vi "Log_WriteLog.vi"(4 "Additional text":string, 6 "All read":string, 8 "error in (no error)":errorcluster, 9 "Response":string, 10 "Command":string, 11 "Log in":refnum<class "Log.lvclass">) -> (0 "error out":errorcluster, 3 "Log out":refnum<class "Log.lvclass">)   [LabVIEW 2024, in "Log.lvclass"]
uses:
  Log.lvclass
  Log.lvclass/Log.ctl
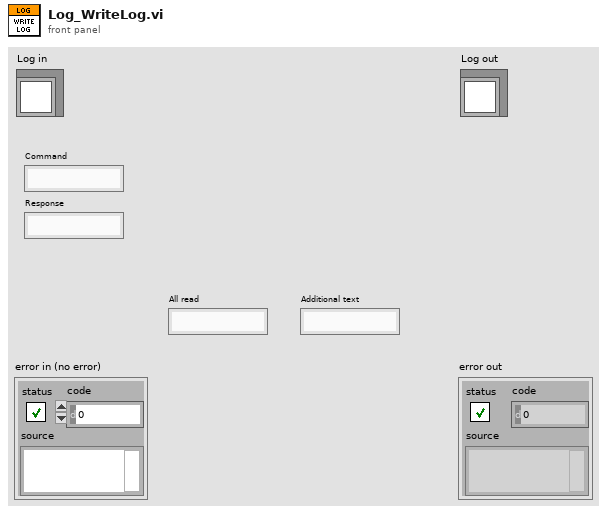
[diagram p1: front panel]
types:
  T1 = enum16{"open", "replace", "create", "open or create", "replace or create", "replace or create with confirmation"}
  T2 = typedef "LVDateTimeRec.ctl" = cluster{"fractional second":dbl, "second":i32, "minute":i32, "hour":i32, "day of month":i32, "month":i32, "year":i32, "day of week":i32, "day of year":i32, "DST":i32}
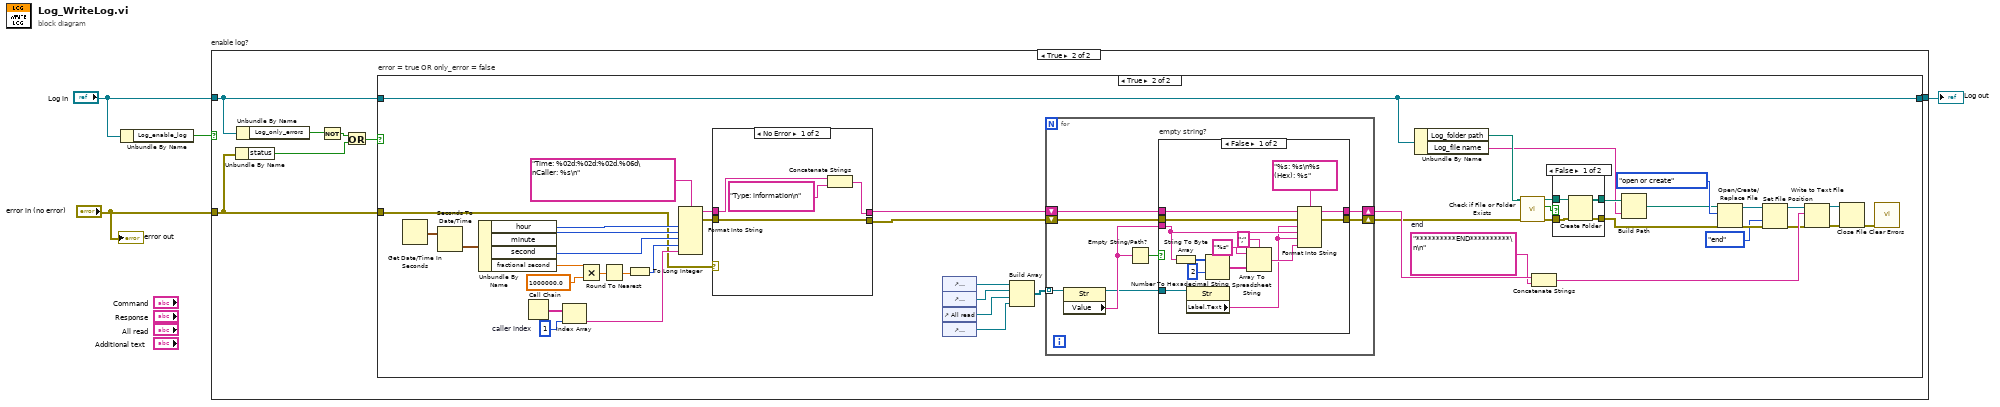
[diagram p0: block diagram]
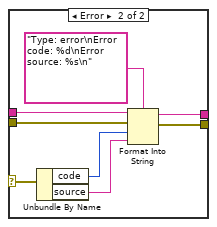
[diagram p6: hidden frame]
diagram:
  n1 = Unbundle By Name("Log in") -> ("Log_enable_log"=w2:bool)
  n2 = case "enable log?" shown="True" w2 {
    tunnel: [w5 w12] -> w4
    tunnel: "Log in" -> [w5 w11]
    tunnel: "error in (no error)" -> [_ w6]
    frame False {
    }
    frame True {
      n3 = Unbundle By Name(w6) -> ("status"=w8:bool)
      n4 = Unbundle By Name(w11) -> ("Log_only_errors"=w10:bool)
      n5 = Not(x=w10) -> (.not. x?=w9:bool)
      n6 = Or(x=w9, y=w8) -> (x .or. y?=w7:bool)
      n7 = case "error = true OR only_error = false" shown="True" w7 {
        tunnel: [w13 w31] -> w12
        tunnel: w11 -> [w13 w31]
        tunnel: w6 -> [_ w41]
        frame False {
        }
        frame True {
          w44 = "**********END**********\n\n"  # end
          w59 = 1  # caller index
          n8 = Get Date/Time In Seconds() -> (seconds since 1Jan1904=w55:timestamp)
          n9 = Seconds To Date/Time(time stamp (now)=w55) -> (date time rec=w47:T2)  [unwired: 1 in]
          n10 = Unbundle By Name(w47) -> ("hour"=w48:i32, "minute"=w49:i32, "second"=w50:i32, "fractional second"=w51:dbl)
          n11 = Call Chain() -> (call chain=w56:string[])
          n12 = Index Array(array=w56, index=w59) -> (element=w46:string)
          n13 = Multiply(x=w51, y=1000000.0) -> (x*y=w52:dbl)
          n14 = Round To Nearest(number=w52) -> (nearest integer value=w53:dbl)
          n15 = To Long Integer(number=w53) -> (32bit integer=w54:i32)
          n16 = Format Into String(format string="Time: %02d:%02d:%02d.%06d\nCaller: %s\n", w48, w49, w50, w54, w46) -> (resulting string=w43:string, error out=w42:errorcluster)  [unwired: 2 in]
          n17 = case shown="No Error" w41 {
            selector: w41 -> [_ w98]
            tunnel: w43 -> [w92 w101]
            tunnel: w42 -> [w93 w100]
            tunnel: [w90 w95] -> w39
            tunnel: [w93 w94] -> w40
            frame No Error {
              n18 = Concatenate Strings(w92, "Type: information\n") -> (w90:string)
            }
            frame Error {
              n19 = Unbundle By Name(w98) -> ("code"=w97:i32, "source"=w96:string)
              n20 = Format Into String(format string="Type: error\nError code: %d\nError source: %s\n", initial string=w101, error in=w100, w97, w96) -> (resulting string=w95:string, error out=w94:errorcluster)
            }
          }
          n21 = control-ref of="Command"() -> (w29:refnum<vi>)
          n22 = control-ref of="Response"() -> (w28:refnum<vi>)
          n23 = control-ref of="All read"() -> (w27:refnum<vi>)
          n24 = control-ref of="Additional text"() -> (w26:refnum<vi>)
          n25 = Build Array(w29, w28, w27, w26) -> (w30:refnum<vi>[])
          n26 = for {
            shift-right: [w63] -> w32
            shift-left: w40 -> [w65]
            shift-right: [w67] -> w45
            shift-left: w39 -> [w64]
            tunnel: w30 -> [w62] mode=indexing
            n27 = property class="Str"(reference=w62) -> (reference out=w60:refnum<vi>, "Value"=w61:string)  [unwired: 1 in, 1 out]
            n28 = Empty String/Path?(string/path=w61) -> (empty?=w66:bool)
            n29 = case "empty string?" shown="False" w66 {
              tunnel: w65 -> [w81 w82]
              tunnel: w64 -> [w80 w83]
              tunnel: [w78 w82] -> w63
              tunnel: [w77 w83] -> w67
              tunnel: w61 -> [w76 _]
              tunnel: w60 -> [w69 _]
              frame False {
                n30 = String To Byte Array(string=w76) -> (unsigned byte array=w75:u8[])
                n31 = property class="Str"(reference=w69) -> ("Label.Text"=w68:string)  [unwired: 1 in, 2 out]
                n32 = Number To Hexadecimal String(1:i16 2 ("width (-)"), 2:w75) -> (0:w73:string[])
                n33 = Array To Spreadsheet String(delimiter (Tab)=";", array=w73, 3:"%s" ("format string")) -> (spreadsheet string=w70:string)
                n34 = Format Into String(format string="%s: %s\n%s (Hex): %s", initial string=w80, error in=w81, w68, w76, w68, w70) -> (resulting string=w77:string, error out=w78:errorcluster)
              }
              frame True {
              }
            }
          }
          n35 = Unbundle By Name(w31) -> ("Log_folder path"=w34:path, "Log_file name"=w33:string)
          n36 = call <vilib>:"Check if File or Folder Exists.vi"("error in (no error)"=w32, "path"=w34) -> ("error out"=w38:errorcluster, "file or folder exists?"=w36:bool, "dup path"=w37:path)  [unwired: 7 in]
          n37 = Concatenate Strings(w45, w44) -> (w25:string)
          n38 = case shown="False" w36 {
            tunnel: w37 -> [w87 w89]
            tunnel: w38 -> [w86 w88]
            tunnel: [w85 w88] -> w22
            tunnel: [w84 w89] -> w35
            frame False {
              n39 = Create Folder(path (use dialog)=w87, error in=w86) -> (created path=w84:path, error out=w85:errorcluster)  [unwired: 1 in, 1 out]
            }
            frame True {
            }
          }
          n40 = Build Path(base path=w35, name or relative path=w33) -> (appended path=w23:path)
          n41 = Open/Create/Replace File(file path (use dialog)=w23, error in=w22, operation (0:open)=T1."open or create") -> (refnum out=w17:refnum<file>, error out=w18:errorcluster)  [unwired: 3 in, 1 out]
          n42 = Set File Position(refnum=w17, from (0:start)=enum16{"start", "end", "current"}."end", error in=w18) -> (refnum out=w15:refnum<file>, error out=w14:errorcluster)  [unwired: 1 in]
          n43 = Write to Text File(file (use dialog)=w15, text=w25, error in=w14) -> (refnum out=w19:refnum<file>, error out=w20:errorcluster)  [unwired: 1 in, 1 out]
          n44 = Close File(refnum=w19, error in=w20) -> (error out=w21:errorcluster)  [unwired: 1 out]
          n45 = call <vilib>:"Clear Errors.vi"("error in (no error)"=w21) -> ()  [unwired: 5 in, 2 out]
        }
      }
    }
  }
  "Log out" <- w4
  "error out" <- "error in (no error)"
